vi "Configure Session.vi"(8 "error in":errorcluster, 11 "Plugin in":refnum<class "DFT_Spectra.lvclass">) -> (0 "error out":errorcluster, 3 "Plugin out":refnum<class "DFT_Spectra.lvclass">)   [LabVIEW 2024, in "DFT_Spectra.lvlib" / "DFT_Spectra.lvclass"]
uses:
  DFT_Spectra.lvclass
  C:/Program Files/National Instruments/LabVIEW 2024/vi.lib/FlexLogger/SDK/PluginSDK.lvlibp/PEFClasses/SDK/Plugin/Plugin.lvclass
  DFT_Spectra Data.ctl
  <vilib>/Analysis/4window.llb/windowTd.ctl
  <vilib>/addons/_NISVFA/_Shared subVIs/Data Objects/Waveforms (DBL)/Waveforms (N Ch).lvclass
  <vilib>/FlexLogger/SDK/PluginSDK.lvlibp/PEFClasses/SDK/Processing Element/Timing Parameters.ctl
  <vilib>/FlexLogger/SDK/PluginSDK.lvlibp/PEFClasses/SDK/Processing Element/Timing Method.ctl
  <vilib>/FlexLogger/SDK/PluginSDK.lvlibp/PEFClasses/SDK/System Interface/Resampling Mode.ctl
  DFT_Spectra.lvclass/DFT_Spectra.ctl
  DFT_Spectra Global.vi
  <vilib>/FlexLogger/SDK/PluginSDK.lvlibp/PEFClasses/SDK/Plugin/ParameterAccess/Read DBL.vi
  <vilib>/FlexLogger/SDK/PluginSDK.lvlibp/PEFClasses/SDK/Plugin/ParameterAccess/Read Enum.vi
  <vilib>/FlexLogger/SDK/PluginSDK.lvlibp/PEFClasses/SDK/Plugin/ParameterAccess/Read I32.vi
  <vilib>/addons/_NISVFA/_Shared subVIs/Data Objects/Data/Data.lvclass
  <vilib>/FlexLogger/SDK/PluginSDK.lvlibp/PEFClasses/SDK/Plugin/Plugin.lvclass
  <vilib>/Utility/LVLibp/NI_PackedLibraryUtility.lvlib
  <vilib>/Analysis/NI_AALPro.lvlib
  <vilib>/FlexLogger/SDK/PluginSDK.lvlibp/PEFClasses/SDK/Processing Element/Processing Element.lvclass
  <vilib>/FlexLogger/SDK/PluginSDK.lvlibp/PEFClasses/SDK/System Interface/System Interface.lvclass
  C:/Program Files/National Instruments/LabVIEW 2024/vi.lib/FlexLogger/SDK/PluginSDK.lvlibp/PEFClasses/SDK/Processing Element/Processing Element.lvclass
  C:/dev/dsb/niflexlogger-plugins/PDK plugins/DFT_Spectra/source/DFT_Spectra.lvclass
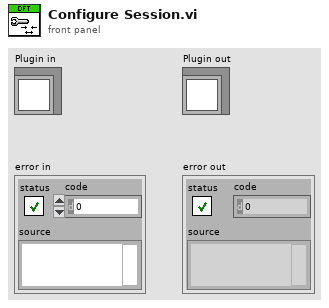
[diagram p1: front panel]
types:
  T1 = cluster{"averaging mode":enum16{"No averaging", "Vector averaging", "RMS averaging", "Peak hold"}, "weighting mode":enum16{"Linear", "Exponential"}, "number of averages":u32}
  T2 = typedef "PluginSDK.lvlibp/System Interface.lvclass/Resampling Mode.ctl" = enum16{"No Resampling", "Custom Rate", "Maximum Rate", "Minimum Rate"}
  T3 = typedef "PluginSDK.lvlibp/Processing Element.lvclass/Timing Parameters.ctl" = cluster{"Timing Method":T4, "Timing Period (ms)":i32}
  T4 = typedef "PluginSDK.lvlibp/Processing Element.lvclass/Timing Method.ctl" = enum16{"Periodic", "Immediate", "On Data Ready", "Triggered"}
  T5 = typedef "DFT_Spectra.lvlib/DFT_Spectra.lvclass/DFT_Spectra Data.ctl" = cluster{"First Time":bool, "Show Results Window":bool, "Show Results Window Clicked":bool, "Window":T6, "overlap":i32, "Block Duration":dbl, "Averaging parameters":cluster{"averaging mode":enum16{"No averaging", "Vector averaging", "RMS averaging", "Peak hold"}, "weighting mode":enum16{"Linear", "Exponential"}, "number of averages":u32}, "buffer out":refnum<data-value>, "Avg Spectra":refnum<vi>, "Spectra UI":refnum<vi>}
  T6 = typedef "NI_AALPro.lvlib/windowTd.ctl" = u32
  T7 = enum16{"No averaging", "Vector averaging", "RMS averaging", "Peak hold"}[]
  T8 = enum16{"No averaging", "Vector averaging", "RMS averaging", "Peak hold"}
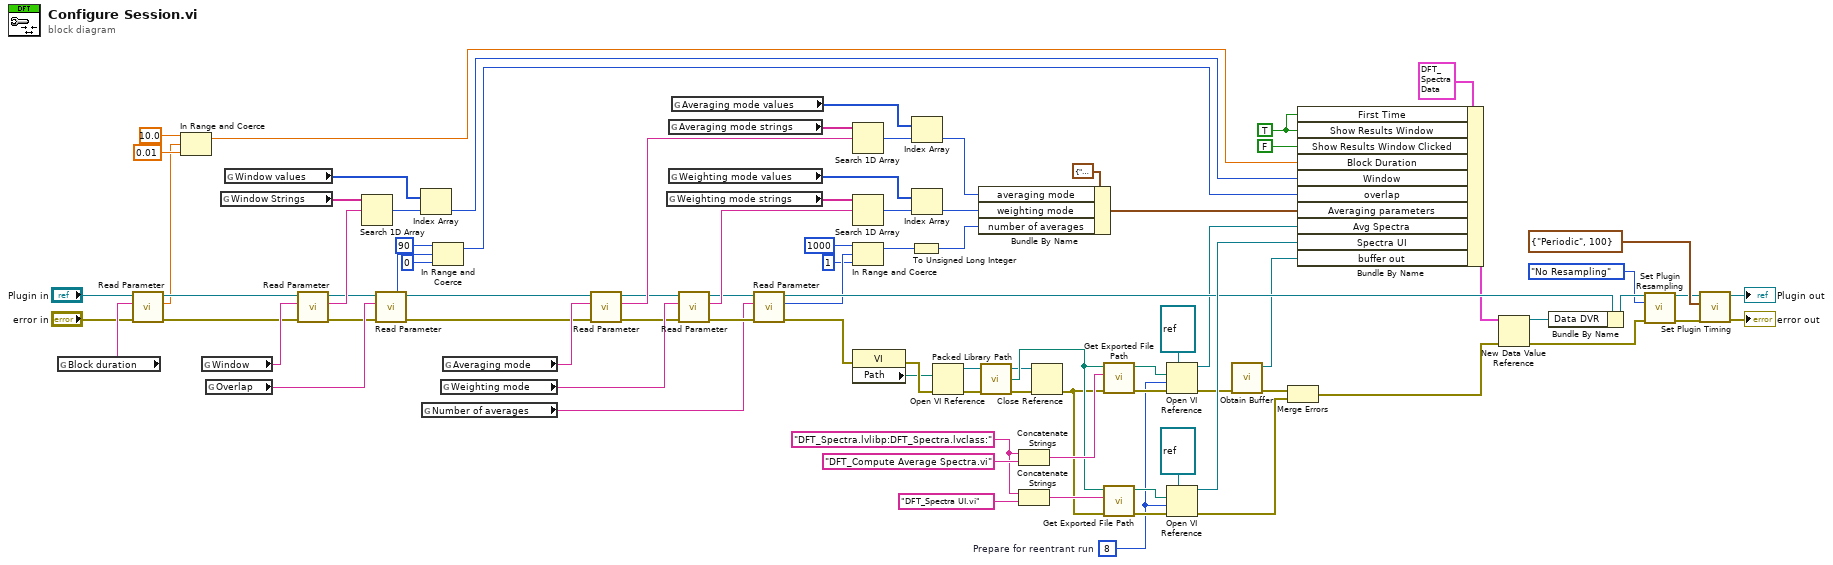
[diagram p0: block diagram]
diagram:
  w20 = "DFT_Spectra.lvlibp:DFT_Spectra.lvclass:" ("qualified name")
  w23 = 8  # Prepare for reentrant run
  w89 = TRUE ("Show Spectrogram Window")
  n1 = global read "DFT_Spectra Global.vi" "Block duration"() -> (w56:string)
  n2 = call-poly <vilib>:"Read Parameter.vi"("error in (no error)"="error in", "Name"=w56, "Plugin in"="Plugin in") -> ("error out"=w52:errorcluster, "Value"=w4:dbl, "Plugin out"=w53:refnum<class "DFT_Spectra.lvclass">)  [unwired: 5 in, 1 out]
  n3 = In Range and Coerce(upper limit=10.0, x=w4, lower limit=0.01) -> (coerced(x)=w3:dbl)  [unwired: 1 out]
  n4 = global read "DFT_Spectra Global.vi" "Window"() -> (w83:string)
  n5 = global read "DFT_Spectra Global.vi" "Overlap"() -> (w67:string)
  n6 = global read "DFT_Spectra Global.vi" "Window Strings"() -> (w84:string[])
  n7 = global read "DFT_Spectra Global.vi" "Window values"() -> (w85:u32[])
  n8 = call-poly <vilib>:"Read Parameter.vi"("error in (no error)"=w52, "Name"=w83, "Plugin in"=w53) -> ("error out"=w50:errorcluster, "Value"=w87:string, "Plugin out"=w51:refnum<class "DFT_Spectra.lvclass">)  [unwired: 4 in, 2 out]
  n9 = Search 1D Array(1D array=w84, element=w87) -> (index of element=w86:i32)  [unwired: 1 in]
  n10 = call-poly <vilib>:"Read Parameter.vi"("error in (no error)"=w50, "Name"=w67, "Plugin in"=w51) -> ("error out"=w48:errorcluster, "Value"=w7:i32, "Plugin out"=w49:refnum<class "DFT_Spectra.lvclass">)  [unwired: 5 in, 1 out]
  n11 = Index Array(array=w85, index=w86) -> (element=w2:u32)
  n12 = global read "DFT_Spectra Global.vi" "Number of averages"() -> (w68:string)
  n13 = In Range and Coerce(upper limit=90, x=w7, lower limit=0) -> (coerced(x)=w1:i32)  [unwired: 1 out]
  n14 = global read "DFT_Spectra Global.vi" "Weighting mode"() -> (w73:string)
  n15 = global read "DFT_Spectra Global.vi" "Averaging mode"() -> (w78:string)
  n16 = call-poly <vilib>:"Read Parameter.vi"("error in (no error)"=w48, "Name"=w78, "Plugin in"=w49) -> ("error out"=w71:errorcluster, "Value"=w82:string, "Plugin out"=w72:refnum<class "DFT_Spectra.lvclass">)  [unwired: 4 in, 2 out]
  n17 = global read "DFT_Spectra Global.vi" "Weighting mode strings"() -> (w74:string[])
  n18 = global read "DFT_Spectra Global.vi" "Averaging mode strings"() -> (w79:string[])
  n19 = global read "DFT_Spectra Global.vi" "Weighting mode values"() -> (w75:enum16{"Linear", "Exponential"}[])
  n20 = global read "DFT_Spectra Global.vi" "Averaging mode values"() -> (w80:T7)
  n21 = call-poly <vilib>:"Read Parameter.vi"("error in (no error)"=w71, "Name"=w73, "Plugin in"=w72) -> ("error out"=w69:errorcluster, "Value"=w77:string, "Plugin out"=w70:refnum<class "DFT_Spectra.lvclass">)  [unwired: 4 in, 2 out]
  n22 = call-poly <vilib>:"Read Parameter.vi"("error in (no error)"=w69, "Name"=w68, "Plugin in"=w70) -> ("error out"=w17:errorcluster, "Value"=w43:i32, "Plugin out"=w47:refnum<class "DFT_Spectra.lvclass">)  [unwired: 5 in, 1 out]
  n23 = Search 1D Array(1D array=w79, element=w82) -> (index of element=w81:i32)  [unwired: 1 in]
  n24 = Search 1D Array(1D array=w74, element=w77) -> (index of element=w76:i32)  [unwired: 1 in]
  n25 = In Range and Coerce(upper limit=1000, x=w43, lower limit=1) -> (coerced(x)=w40:i32)  [unwired: 1 out]
  n26 = property class="VI"(error in=w17) -> (error out=w31:errorcluster, "Path"=w16:path)  [unwired: 1 in, 1 out]
  n27 = To Unsigned Long Integer(number=w40) -> (unsigned 32bit integer=w63:u32)
  n28 = Index Array(array=w80, index=w81) -> (element=w65:T8)
  n29 = Index Array(array=w75, index=w76) -> (element=w64:enum16{"Linear", "Exponential"})
  n30 = Open VI Reference(vi path=w16, error in (no error)=w31) -> (vi reference=w29:refnum<vi>, error out=w30:errorcluster)  [unwired: 4 in]
  n31 = Bundle By Name(cluster=T1 {"averaging mode"=enum."No averaging", "weighting mode"=enum."Linear", "number of averages"=0} ("Averaging parameters"), "averaging mode"=w65, "weighting mode"=w64, "number of averages"=w63) -> (w28:T1)
  n32 = call <vilib>:"Packed Library Path.vi"("error in (no error)"=w30, "vi reference"=w29) -> ("error out"=w14:errorcluster, "packed library path"=w15:path, "vi reference out"=w12:refnum<vi>)  [unwired: 1 in]
  n33 = Concatenate Strings(w20, "DFT_Compute Average Spectra.vi" ("qualified name")) -> (w21:string)
  n34 = Concatenate Strings(w20, "DFT_Spectra UI.vi" ("qualified name")) -> (w18:string)
  n35 = Close Reference(reference=w12, error in (no error)=w14) -> (error out=w13:errorcluster)
  n36 = call <vilib>:"Get Exported File Path.vi"("error in (no error)"=w13, "qualified name"=w21, "packed library path"=w15) -> ("error out"=w34:errorcluster, "path"=w33:path)  [unwired: 7 in]
  n37 = call <vilib>:"Get Exported File Path.vi"("error in (no error)"=w13, "qualified name"=w18, "packed library path"=w15) -> ("error out"=w36:errorcluster, "path"=w37:path)  [unwired: 7 in]
  n38 = Open VI Reference(type specifier VI Refnum (for type only)=refnum<vi> refnum, vi path=w33, options=w23, error in (no error)=w34) -> (vi reference=w25:refnum<vi>, error out=w27:errorcluster)  [unwired: 2 in]
  n39 = Open VI Reference(type specifier VI Refnum (for type only)=refnum<vi> refnum, vi path=w37, options=w23, error in (no error)=w36) -> (vi reference=w57:refnum<vi>, error out=w46:errorcluster)  [unwired: 2 in]
  n40 = call <vilib>:"Obtain Buffer.vi"("error in (no error)"=w27) -> ("error out"=w26:errorcluster, "buffer out"=w35:refnum<data-value>)  [unwired: 9 in]
  n41 = Merge Errors(w26, w46) -> (w11:errorcluster)
  n42 = Bundle By Name(cluster=T5 {"First Time"=FALSE, "Show Results Window"=FALSE, "Show Results Window Clicked"=FALSE, "Window"=0, "overlap"=0, "Block Duration"=0.0, "Averaging parameters"={"averaging mode"=enum."No averaging", "weighting mode"=enum."Linear", "number of averages"=0}, "buffer out"=refnum, "Avg Spectra"=refnum, "Spectra UI"=refnum} ("Data"), "First Time"=w89, "Show Results Window"=w89, "Show Results Window Clicked"=FALSE ("Show Spectrogram Window"), "Block Duration"=w3, "Window"=w2, "overlap"=w1, "Averaging parameters"=w28, "Avg Spectra"=w25, "Spectra UI"=w57, "buffer out"=w35) -> (w39:T5)
  n43 = New Data Value Reference(data value=w39, error in=w11) -> (data value reference=w62:refnum<data-value>, error out=w10:errorcluster)
  n44 = Bundle By Name(cluster=w47, "Data DVR"=w62) -> (w59:refnum<class "DFT_Spectra.lvclass">)
  n45 = call <vilib>:"Set Plugin Resampling.vi"("Plugin in"=w59, "Resampling Mode"=Resampling_Mode."No Resampling", "error in (no error)"=w10) -> ("Plugin out"=w45:refnum<class "DFT_Spectra.lvclass">, "error out"=w44:errorcluster)  [unwired: 11 in]
  n46 = call <vilib>:"Set Plugin Timing.vi"("error in (no error)"=w44, "Timing Parameters"=T3 {"Timing Method"=enum."Periodic", "Timing Period (ms)"=100}, "Plugin in"=w45) -> ("error out"=→"error out":errorcluster, "Plugin out"=→"Plugin out":refnum<class "DFT_Spectra.lvclass">)  [unwired: 7 in]
